vi "xeva-getData.vi"(3 "error in (no error)":errorcluster, 5 "xeva-camref-in":T1=refnum) -> (0 "error out":errorcluster, 1 "xeva-data":u16[](array[numeric]), 2 "xeva-camref-out":T1)   [LabVIEW 2015]
doc: "This example shows how to open the camera, grab frames and display them on the control-panel. To get a better visualisation the histogram is spread."
uses:
  <vilib>/Xenics Infrared Solutions/Xeneth LabVIEW API/VIs/Controls/Camara.ctl
  <vilib>/Xenics Infrared Solutions/Xeneth LabVIEW API/VIs/Controls/FrameType.ctl
  <vilib>/Xenics Infrared Solutions/Xeneth LabVIEW API/Xeneth.lvlib
panel:
  # "This example shows how to open the camera, grab frames and display them on the control-panel. \nTo get a better visualisation the histogram is spread. The picture can although be acquired using GetPicture.vi. \nThe code inside the while-loop essentially the same. Here a 16 Bit Camera is assumed."
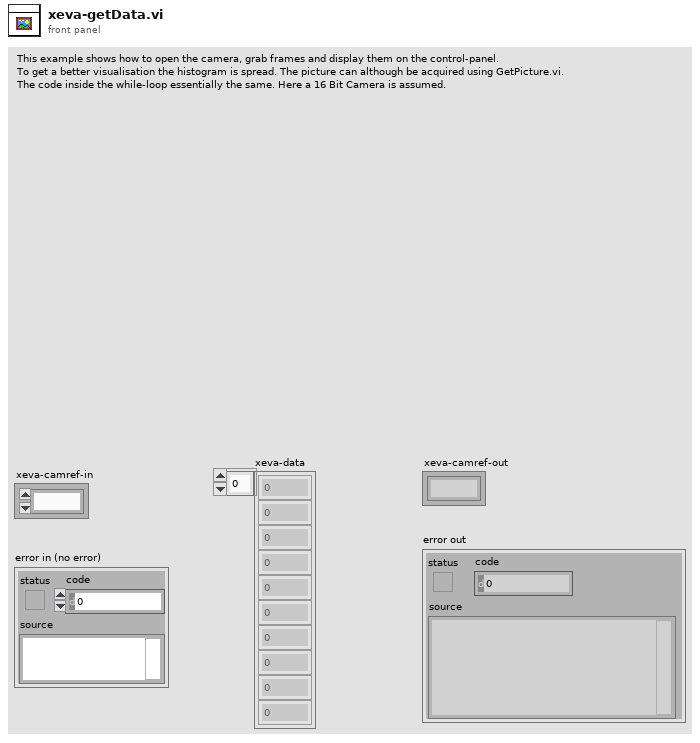
[diagram p1: front panel]
types:
  T1 = typedef "Xeneth.lvlib/Camara.ctl" = refnum<k1>
  T2 = typedef "Xeneth.lvlib/FrameType.ctl" = u32
  T3 = enum16{"big-endian, network order", "native, host order", "little-endian"}
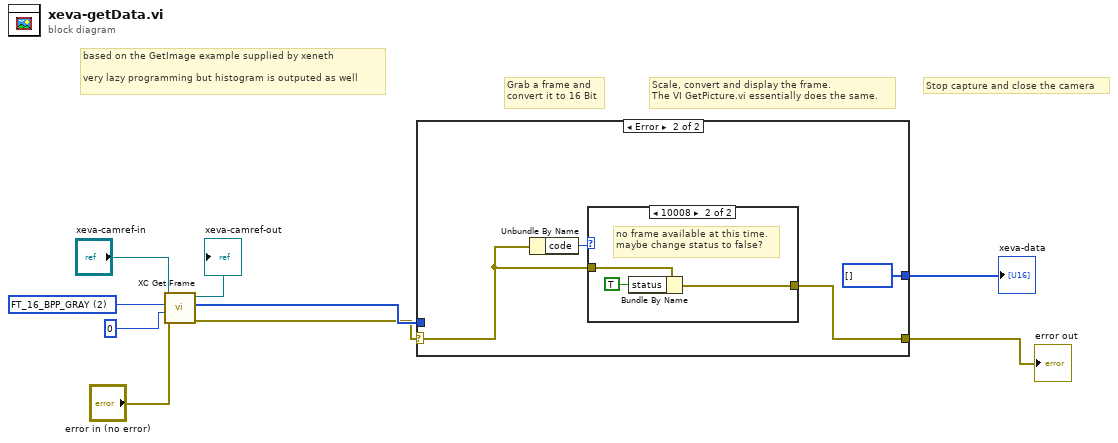
[diagram p0: block diagram]
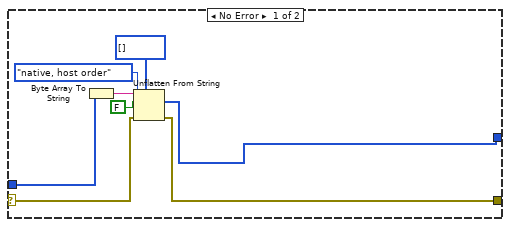
[diagram p2: hidden frame]
diagram:
  w9 = T2 2 items=["FT_NATIVE", "FT_8_BPP_GRAY", "FT_16_BPP_GRAY", "FT_32_BPP_GRAY", "FT_32_BPP_RGBA", "FT_32_BPP_RGB", "FT_32_BPP_BGRA", "FT_32_BPP_BGR"] ("type")
  # "based on the GetImage example supplied by xeneth\n\nvery lazy programming but histogram is outputed as well"
  # "Grab a frame and \nconvert it to 16 Bit"
  # "Scale, convert and display the frame.\nThe VI GetPicture.vi essentially does the same."
  # "Stop capture and close the camera"
  n1 = call <vilib>:"XC Get Frame.vi"("error in (no error)"="error in (no error)", "uFlags"=0, "type"=w9, "Cam Ref 2"="xeva-camref-in") -> ("error out"=w3:errorcluster, "buffer"=w8:u8[], "Cam Ref Out"=→"xeva-camref-out":T1)  [unwired: 5 in]
  n2 = case shown="Error" w3 {
    selector: w3 -> [w11 w19]
    tunnel: w8 -> [w13 _]
    tunnel: [w12 w18] -> w4
    tunnel: [w10 u16[] [] ("Data")] -> w2
    frame No Error {
      n3 = Byte Array To String(unsigned byte array=w13) -> (string=w17:string)
      n4 = Unflatten From String(type=u16[] [] ("Data"), binary string=w17, data includes array or string size? (T)=FALSE, byte order (0:big-endian, network order)=T3."native, host order", error in (no error)=w11) -> (value=w10:u16[], error out=w12:errorcluster)  [unwired: 1 out]
    }
    frame Error {
      n5 = Unbundle By Name(w19) -> ("code"=w20:i32)
      n6 = case shown="10008" w20 {
        tunnel: w19 -> [w22 w25]
        tunnel: [w22 w24] -> w18
        frame Default {
        }
        frame 10008 {
          # "no frame available at this time.\nmaybe change status to false?"
          n7 = Bundle By Name(cluster=w25, "status"=TRUE) -> (w24:errorcluster)
        }
      }
    }
  }
  "error out" <- w4
  "xeva-data" <- w2
